vi "Sound Signal.vi"(8 "error in (no error)":errorcluster, 11 "Car in":refnum<class "Car.lvclass">) -> (0 "error out":errorcluster, 3 "Car out":refnum<class "Car.lvclass">)   [LabVIEW 2019, in "Car.lvclass"]
uses:
  Car.lvclass
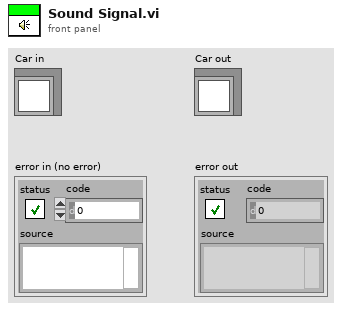
[diagram p1: front panel]
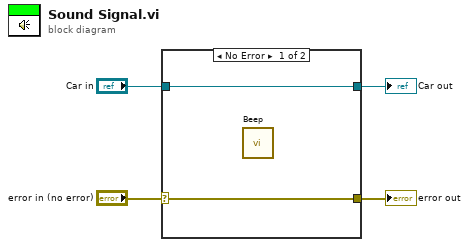
[diagram p0: block diagram]
diagram:
  n1 = case shown="No Error" "error in (no error)" {
    selector: "error in (no error)" -> [w5 w7]
    tunnel: "Car in" -> [w6 w8]
    tunnel: [w6 w8] -> w2
    tunnel: [w5 w7] -> w1
    frame No Error {
      n2 = call <vilib>:"Beep.vi"() -> ()  [unwired: 12 in]
    }
    frame Error {
    }
  }
  "error out" <- w1
  "Car out" <- w2
